vi "prepare camera buffer.vi"(7 "buffer page size":u32, 9 "frame #":u32, 10 "frame height":u16, 11 "frame width":u16) -> (1 "buffer pointers":u64[](array[numeric]), 3 "buffer array":T1[](array[typedef]))   [LabVIEW 2015]
uses:
  <vilib>/vision/Image Controls.llb/IMAQ Image.ctl
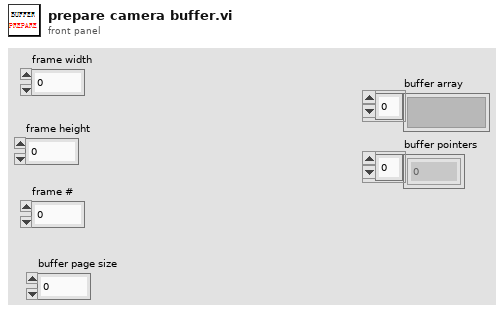
[diagram p1: front panel]
types:
  T1 = typedef "IMAQ Image.ctl" = refnum<image>
  T2 = enum32{"Map Pixel Pointer", "Unmap Pixel Pointer", "Get Pixels Infos"}
  T3 = typedef "Image Type" = u32
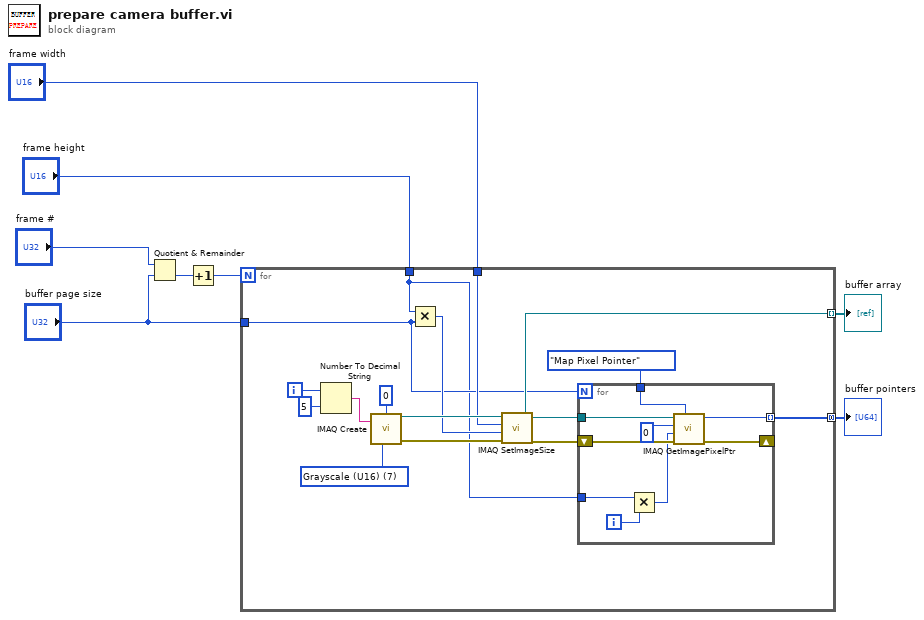
[diagram p0: block diagram]
diagram:
  n1 = Quotient & Remainder(x="frame #", y="buffer page size") -> (floor(x/y)=w7:u32)  [unwired: 1 out]
  n2 = Increment(x=w7) -> (x+1=w6:u32)
  n3 = for {
    N: w6 -> [_]
    tunnel: [w13] -> w2 mode=indexing
    tunnel: [w18] -> w1 mode=concatenating
    tunnel: "frame height" -> [w9]
    tunnel: "buffer page size" -> [w10]
    tunnel: "frame width" -> [w11]
    i -> [w23]
    w15 = T3 7 items=["Grayscale (U8)", "Grayscale (I16)", "Grayscale (SGL)", "Complex (CSG)", "RGB (U32)", "HSL (U32)", "RGB (U64)", "Grayscale (U16)"] ("Image Type")
    n4 = Number To Decimal String(number=w23, width (-)=i16 5) -> (decimal integer string=w21:string)
    n5 = call "IMAQ Create"("Border Size"=0, "Image Name"=w21, "Image Type"=w15) -> ("New Image"=w17:T1, "error out"=w16:errorcluster)  [unwired: 2 in]
    n6 = Multiply(x=w9, y=w10) -> (x*y=w12:u32)
    n7 = call "IMAQ SetImageSize"("error in (no error)"=w16, "Y Resolution"=w12, "X Resolution"=w11, "Image"=w17) -> ("error out"=w14:errorcluster, "Image Out"=w13:T1)  [unwired: 1 in]
    n8 = for {
      N: w10 -> [_]
      tunnel: T2."Map Pixel Pointer" ("Function") -> [w32]
      tunnel: [w30] -> w18 mode=indexing
      tunnel: w13 -> [w28]
      shift-right: [w27] -> _
      shift-left: w14 -> [w29]
      tunnel: w9 -> [w24]
      i -> [w26]
      n9 = Multiply(x=w24, y=w26) -> (x*y=w25:i32)
      n10 = call "IMAQ GetImagePixelPtr"("Function"=w32, "error in (no error)"=w29, "Y Coordinate"=w25, "X Coordinate"=0, "Image"=w28) -> ("error out"=w27:errorcluster, "Pixel Pointer out"=w30:u64)  [unwired: 1 in, 4 out]
    }
  }
  "buffer array" <- w2
  "buffer pointers" <- w1
